vi "TCP-KO-Send Command.vi"(0 "connection ID":refnum<k5>, 7 "Command":string, 9 "timeout (ms)":i32=5000, 11 "error in (no error)":errorcluster, 12 "fast response":bool) -> (4 "connection ID out":refnum<k5>, 15 "error out":errorcluster)   [LabVIEW 2020]
panel:
  out "result":i32
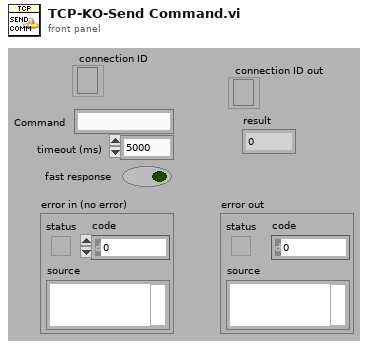
[diagram p1: front panel]
types:
  T1 = enum16{"Standard", "Buffered", "CRLF", "Immediate"}
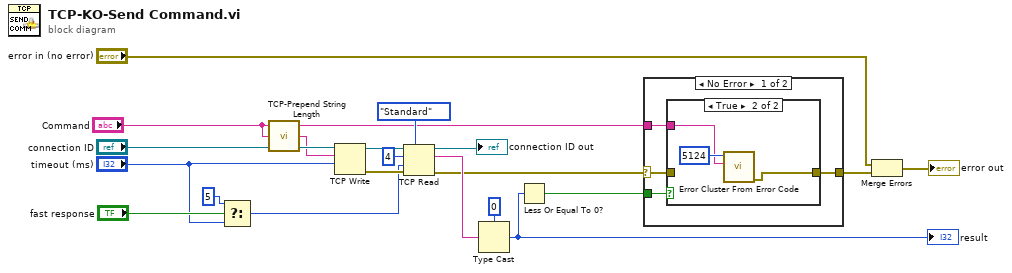
[diagram p0: block diagram]
diagram:
  n1 = Select(t=5 ("timeout ms (25000)"), s="fast response", f="timeout (ms)") -> (s? t:f=w7:i32)
  n2 = call "TCP-Prepend String Length.vi"("Command"="Command") -> ("String"=w1:string)  [unwired: 4 in]
  n3 = TCP Write(connection ID="connection ID", data in=w1, 9:"timeout (ms)") -> (connection ID out=w20:refnum<k5>, error out=w11:errorcluster)  [unwired: 1 in, 1 out]
  n4 = TCP Read(connection ID=w20, bytes to read=4, error in (no error)=w11, 7:T1."Standard" ("mode (standard)"), 9:w7) -> (connection ID out=→"connection ID out":refnum<k5>, data out=w19:string, error out=w10:errorcluster)
  n5 = Type Cast(type=0, x=w19) -> (*(type *) &x=w5:i32)
  "result" <- w5
  n6 = Less Or Equal To 0?(x=w5) -> (x <= 0?=w17:bool)
  n7 = case shown="No Error" w10 {
    selector: w10 -> [w22 w29]
    tunnel: w17 -> [w24 _]
    tunnel: [w23 w29] -> w16
    tunnel: "Command" -> [w21 _]
    frame No Error {
      n8 = case shown="True" w24 {
        tunnel: [w25 w26] -> w23
        tunnel: w22 -> [w25 _]
        tunnel: w21 -> [_ w27]
        frame False {
        }
        frame True {
          n9 = call <vilib>:"Error Cluster From Error Code.vi"("error message (\"\")"=w27, "error code (0)"=5124) -> ("error out"=w26:errorcluster)  [unwired: 7 in]
        }
      }
    }
    frame Error {
    }
  }
  n10 = Merge Errors("error in (no error)", w16) -> (→"error out":errorcluster)
